vi "Make Option String.vi"(8 "error in":errorcluster, 10 "RTG API Options":T1={"Local?"=enum."Local", "Cal"={"enable internal loopback  "=FALSE, "enable overwrite cal data  "=FALSE, "enable save cal data           "=FALSE, "disable self cal range          "=FALSE}, "Remote"={"ip address"="", "port"="50052", "certificate path"=path "", "timeout (ms)"=15000}, "ini path"=path ""}, 11 "instrument names":string[](array[string])) -> (0 "error out":errorcluster, 3 "option string":string)   [LabVIEW 2020, in "RTG Examples.lvlib"]
uses:
  RTG Examples.lvlib
  <vilib>/RTG/API/ip/rtg-options/RTG Options.lvclass
  <vilib>/RTG/API/ip/local-api/NI-RTG Local API.lvclass
  <vilib>/RTG/API/ip/rtg-options/protected/Set Option - API Implementation.vi
  <vilib>/RTG/API/ip/rtg-options/protected/Set Option - Self Cal Range Disable.vi
  <vilib>/RTG/API/ip/rtg-options/protected/Set Option - INI File Path.vi
  <vilib>/RTG/API/ip/rtg-options/protected/Set Option - Internal Loopback Enable.vi
  <vilib>/RTG/API/remote/NI-RTG gRPC Client.lvclass
  <vilib>/RTG/API/ip/rtg-options/protected/Set Option - Timeout.vi
  <vilib>/RTG/API/ip/rtg-options/protected/Set Option - IP Address.vi
  <vilib>/RTG/API/ip/rtg-options/protected/Set Option - Port.vi
  <vilib>/RTG/API/ip/rtg-options/protected/Set Option - Certificate Path.vi
  <vilib>/RTG/API/ip/rtg-options/protected/Set Option - Overwrite Calibration Enable.vi
  <vilib>/RTG/API/ip/rtg-options/protected/Set Option - Save Calibration Enable.vi
  C:/Program Files/National Instruments/LabVIEW 2020/vi.lib/RTG/API/interface/NI-RTG Interface.lvclass
  C:/Program Files/National Instruments/LabVIEW 2020/vi.lib/RTG/API/ip/local-api/NI-RTG Local API.lvclass
  C:/Program Files/National Instruments/LabVIEW 2020/vi.lib/RTG/API/remote/NI-RTG gRPC Client.lvclass
  Options - Remote.ctl
  Options - API Mode.ctl
  Options - Calibration.ctl
  Controls/Clust/RTG API Clust.ctl
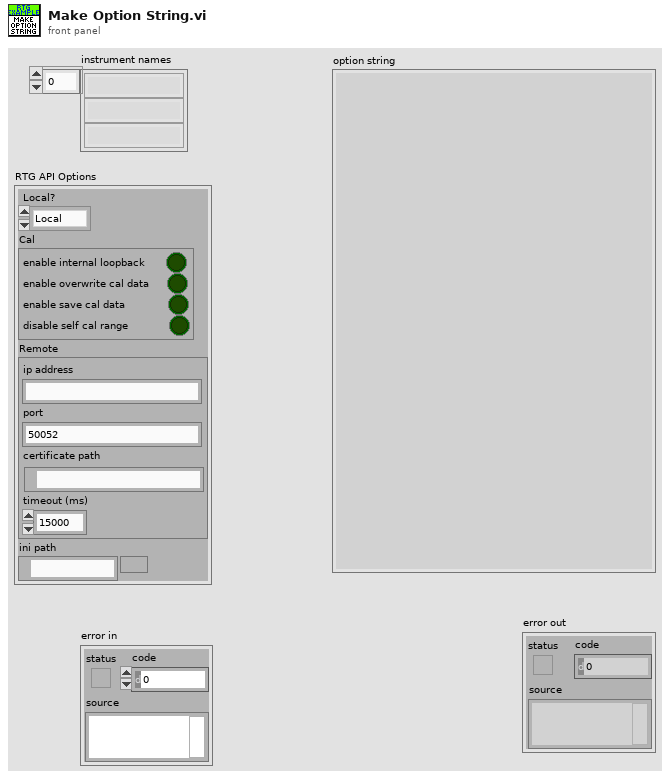
[diagram p1: front panel]
types:
  T1 = typedef "RTG API Clust.ctl" = cluster{"Local?":T2, "Cal":T3, "Remote":T4, "ini path":path}
  T2 = typedef "RTG Examples.lvlib/Options - API Mode.ctl" = enum16{"Local", "Remote"}
  T3 = typedef "RTG Examples.lvlib/Options - Calibration.ctl" = cluster{"enable internal loopback  ":bool, "enable overwrite cal data  ":bool, "enable save cal data           ":bool, "disable self cal range          ":bool}
  T4 = typedef "RTG Examples.lvlib/Options - Remote.ctl" = cluster{"ip address":string, "port":string, "certificate path":path, "timeout (ms)":i32}
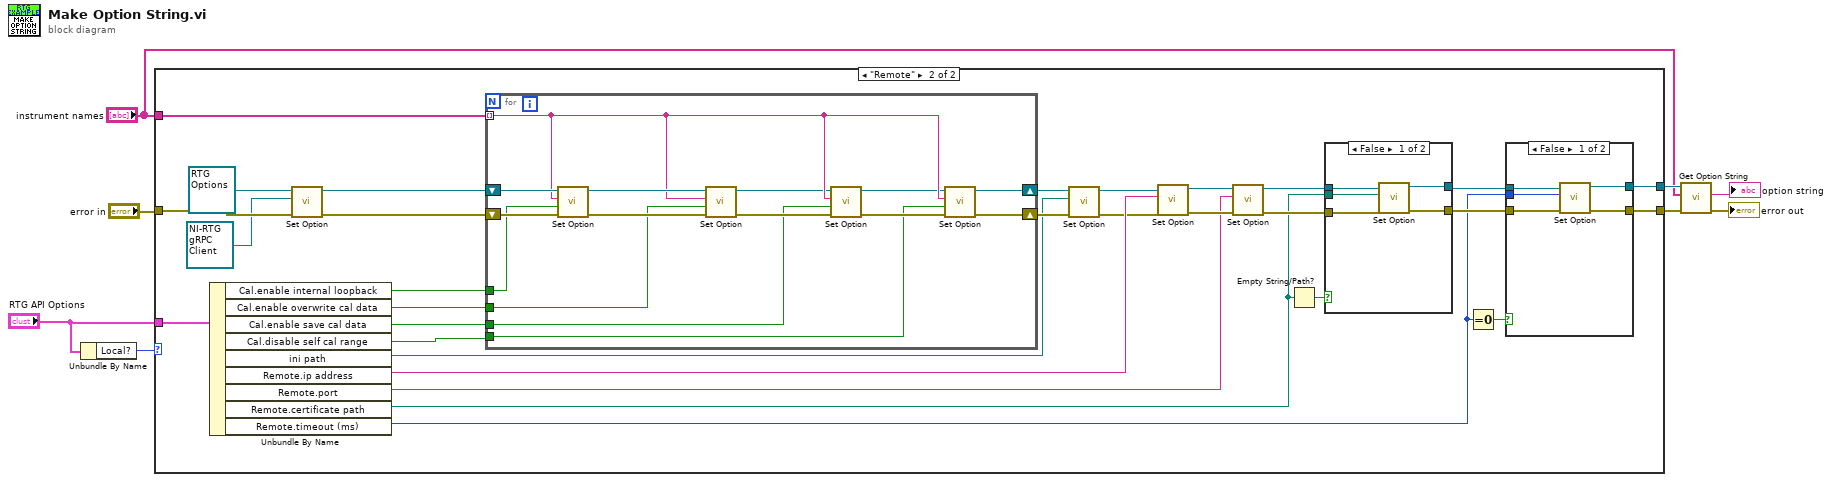
[diagram p0: block diagram]
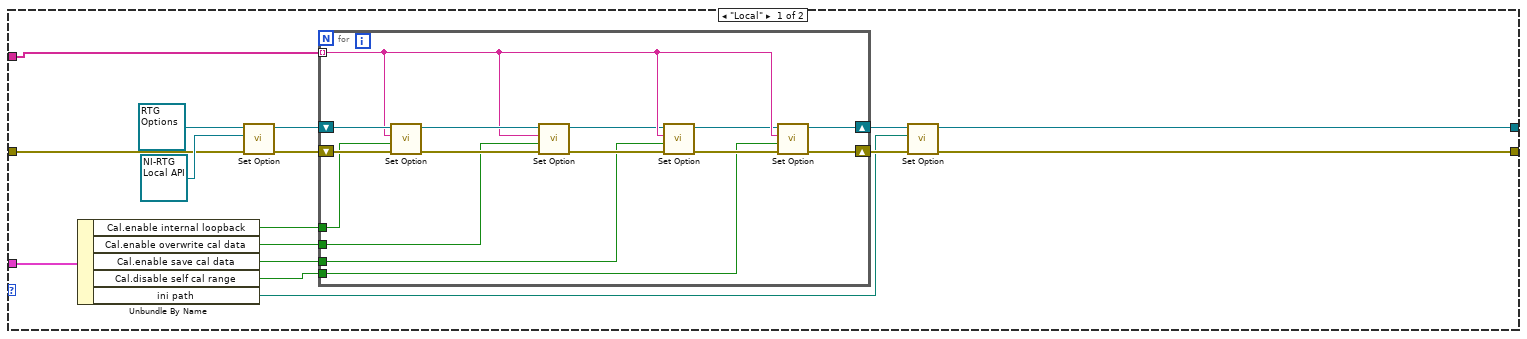
[diagram p2: hidden frame]
diagram:
  n1 = Unbundle By Name("RTG API Options") -> ("Local?"=w7:T2)
  n2 = case shown="\"Remote\"" w7 {
    tunnel: [w20 w46] -> w5
    tunnel: [w21 w45] -> w6
    tunnel: "error in" -> [w22 w60]
    tunnel: "instrument names" -> [w15 w53]
    tunnel: "RTG API Options" -> [w19 w55]
    frame "Local" {
      n3 = Unbundle By Name(w19) -> ("Cal.enable internal loopback"=w13:bool, "Cal.enable overwrite cal data"=w12:bool, "Cal.enable save cal data"=w11:bool, "Cal.disable self cal range"=w10:bool, "ini path"=w9:path)
      n4 = call-poly <vilib>:"Set Option.vi"("error in"=w22, "rtg api implementation"=refnum<class "NI-RTG Local API.lvclass"> refnum ("NI-RTG Local API.lvclass"), "RTG Option String in"=refnum<class "RTG Options.lvclass"> refnum ("RTG Options v1.lvlib:RTG Options.lvclass")) -> ("error out"=w14:errorcluster, "RTG Option String out"=w18:refnum<class "RTG Options.lvclass">)  [unwired: 7 in]
      n5 = for {
        shift-right: [w25] -> w17
        shift-left: w18 -> [w39]
        shift-right: [w33] -> w16
        shift-left: w14 -> [w38]
        tunnel: w15 -> [w32] mode=indexing
        tunnel: w13 -> [w29]
        tunnel: w12 -> [w28]
        tunnel: w11 -> [w27]
        tunnel: w10 -> [w26]
        n6 = call-poly <vilib>:"Set Option.vi"("error in"=w38, "enable"=w29, "device name (\"\":all)"=w32, "RTG Option String in"=w39) -> ("error out"=w36:errorcluster, "RTG Option String out"=w37:refnum<class "RTG Options.lvclass">)  [unwired: 6 in]
        n7 = call-poly <vilib>:"Set Option.vi"("error in"=w36, "enable"=w28, "device name (\"\":all)"=w32, "RTG Option String in"=w37) -> ("error out"=w35:errorcluster, "RTG Option String out"=w30:refnum<class "RTG Options.lvclass">)  [unwired: 6 in]
        n8 = call-poly <vilib>:"Set Option.vi"("error in"=w35, "enable"=w27, "device name (\"\":all)"=w32, "RTG Option String in"=w30) -> ("error out"=w34:errorcluster, "RTG Option String out"=w31:refnum<class "RTG Options.lvclass">)  [unwired: 6 in]
        n9 = call-poly <vilib>:"Set Option.vi"("error in"=w34, "disable"=w26, "device name (\"\":all)"=w32, "RTG Option String in"=w31) -> ("error out"=w33:errorcluster, "RTG Option String out"=w25:refnum<class "RTG Options.lvclass">)  [unwired: 6 in]
      }
      n10 = call-poly <vilib>:"Set Option.vi"("error in"=w16, "ini file path"=w9, "RTG Option String in"=w17) -> ("error out"=w21:errorcluster, "RTG Option String out"=w20:refnum<class "RTG Options.lvclass">)  [unwired: 7 in]
    }
    frame "Remote" {
      n11 = Unbundle By Name(w55) -> ("Cal.enable internal loopback"=w43:bool, "Cal.enable overwrite cal data"=w42:bool, "Cal.enable save cal data"=w41:bool, "Cal.disable self cal range"=w40:bool, "ini path"=w54:path, "Remote.ip address"=w51:string, "Remote.port"=w49:string, "Remote.certificate path"=w48:path, "Remote.timeout (ms)"=w47:i32)
      n12 = call-poly <vilib>:"Set Option.vi"("error in"=w60, "rtg api implementation"=refnum<class "NI-RTG gRPC Client.lvclass"> refnum ("NI-RTG gRPC Client.lvclass"), "RTG Option String in"=refnum<class "RTG Options.lvclass"> refnum ("RTG Options v1.lvlib:RTG Options.lvclass")) -> ("error out"=w56:errorcluster, "RTG Option String out"=w57:refnum<class "RTG Options.lvclass">)  [unwired: 7 in]
      n13 = for {
        shift-right: [w70] -> w59
        shift-left: w57 -> [w84]
        shift-right: [w78] -> w58
        shift-left: w56 -> [w83]
        tunnel: w53 -> [w77] mode=indexing
        tunnel: w43 -> [w74]
        tunnel: w42 -> [w73]
        tunnel: w41 -> [w72]
        tunnel: w40 -> [w71]
        n14 = call-poly <vilib>:"Set Option.vi"("error in"=w83, "enable"=w74, "device name (\"\":all)"=w77, "RTG Option String in"=w84) -> ("error out"=w81:errorcluster, "RTG Option String out"=w82:refnum<class "RTG Options.lvclass">)  [unwired: 6 in]
        n15 = call-poly <vilib>:"Set Option.vi"("error in"=w81, "enable"=w73, "device name (\"\":all)"=w77, "RTG Option String in"=w82) -> ("error out"=w80:errorcluster, "RTG Option String out"=w75:refnum<class "RTG Options.lvclass">)  [unwired: 6 in]
        n16 = call-poly <vilib>:"Set Option.vi"("error in"=w80, "enable"=w72, "device name (\"\":all)"=w77, "RTG Option String in"=w75) -> ("error out"=w79:errorcluster, "RTG Option String out"=w76:refnum<class "RTG Options.lvclass">)  [unwired: 6 in]
        n17 = call-poly <vilib>:"Set Option.vi"("error in"=w79, "disable"=w71, "device name (\"\":all)"=w77, "RTG Option String in"=w76) -> ("error out"=w78:errorcluster, "RTG Option String out"=w70:refnum<class "RTG Options.lvclass">)  [unwired: 6 in]
      }
      n18 = call-poly <vilib>:"Set Option.vi"("error in"=w58, "ini file path"=w54, "RTG Option String in"=w59) -> ("error out"=w50:errorcluster, "RTG Option String out"=w52:refnum<class "RTG Options.lvclass">)  [unwired: 7 in]
      n19 = call-poly <vilib>:"Set Option.vi"("error in"=w50, "ip address"=w51, "RTG Option String in"=w52) -> ("error out"=w67:errorcluster, "RTG Option String out"=w68:refnum<class "RTG Options.lvclass">)  [unwired: 7 in]
      n20 = call-poly <vilib>:"Set Option.vi"("error in"=w67, "port"=w49, "RTG Option String in"=w68) -> ("error out"=w65:errorcluster, "RTG Option String out"=w66:refnum<class "RTG Options.lvclass">)  [unwired: 7 in]
      n21 = Empty String/Path?(string/path=w48) -> (empty?=w64:bool)
      n22 = case shown="False" w64 {
        tunnel: w66 -> [w96 w98]
        tunnel: w65 -> [w95 w97]
        tunnel: [w94 w98] -> w63
        tunnel: [w93 w97] -> w62
        tunnel: w48 -> [w92 _]
        frame False {
          n23 = call-poly <vilib>:"Set Option.vi"("error in"=w95, "certificate path"=w92, "RTG Option String in"=w96) -> ("error out"=w93:errorcluster, "RTG Option String out"=w94:refnum<class "RTG Options.lvclass">)  [unwired: 7 in]
        }
        frame True {
        }
      }
      n24 = Equal To 0?(x=w47) -> (x = 0?=w61:bool)
      n25 = case shown="False" w61 {
        tunnel: w63 -> [w89 w91]
        tunnel: [w88 w91] -> w46
        tunnel: [w87 w90] -> w45
        tunnel: w62 -> [w86 w90]
        tunnel: w47 -> [w85 _]
        frame False {
          n26 = call-poly <vilib>:"Set Option.vi"("error in"=w86, "timeout (ms)"=w85, "RTG Option String in"=w89) -> ("error out"=w87:errorcluster, "RTG Option String out"=w88:refnum<class "RTG Options.lvclass">)  [unwired: 7 in]
        }
        frame True {
        }
      }
    }
  }
  n27 = call <vilib>:"Get Option String.vi"("error in"=w6, "device names (all)"="instrument names", "RTG Options in"=w5) -> ("error out"=→"error out":errorcluster, "option string"=→"option string":string)  [unwired: 6 in, 1 out]
